vi "Send Actuator Setpoint.vi"(8 "error in (no error)":errorcluster, 10 "SlewFlag":bool, 11 "Model in":refnum<class "Model.lvclass">) -> (0 "error out":errorcluster, 3 "Model out":refnum<class "Model.lvclass">)   [LabVIEW 2016]
uses:
  Common_RT_FAILC/FAILC/FAILC.lvclass
  Modbus/DesktopModbus/DesktopModbus.lvclass
  Model.lvclass
  C:/CODE/ts_HPMT/Common_RT_ILC/ILC/ILC.lvclass
  C:/CODE/ts_HPMT/Common_RT_Modbus/IModbus/IModbus.lvclass
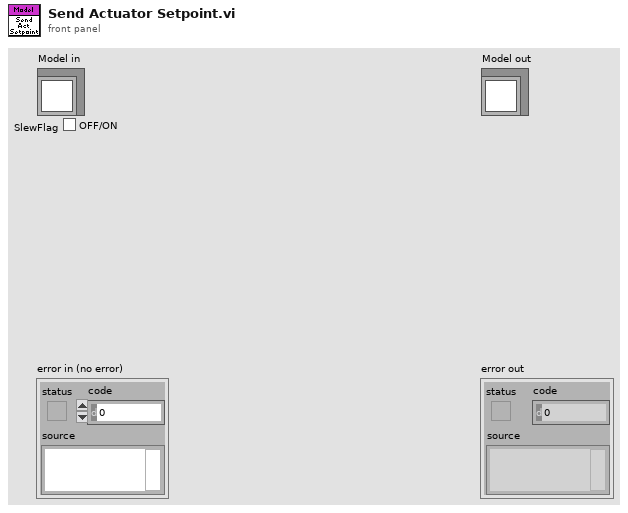
[diagram p1: front panel]
types:
  T1 = typedef "RTHPILC.lvlib/HPData.ctl" = cluster{"Constants":T2, "Command":T3, "Telemetry":T4, "Responses":T5, "Timings":T7}
  T2 = typedef "RTHPILC.lvlib/HPConstants.ctl" = cluster{"ID":i16}
  T3 = typedef "RTHPILC.lvlib/HPCommand.ctl" = cluster{"AxialSetPoint":i32, "LateralSetPoint":i32, "AxialBoosterValveGain":sgl, "LateralBoosterValveGain":sgl}
  T4 = typedef "RTHPILC.lvlib/HPTelemetry.ctl" = cluster{"ILCFault":bool, "BroadcastCounter":u8, "AxialLoadCellForce":sgl, "LateralLoadCellForce":sgl, "AxialBoosterValveGain":sgl, "LateralBoosterValveGain":sgl}
  T5 = typedef "RTHPILC.lvlib/HPResponses.ctl" = cluster{"BoosterValveGain":T6, "ReadBoosterValveGain":T6, "SetForce":T6, "ForceAndStatus":T6}
  T6 = typedef "RTModbus.lvlib/ExceptionCodes.ctl" = u16
  T7 = typedef "RTHPILC.lvlib/HPTimings.ctl" = cluster{"BroadcastSetForce":u32, "BoosterValveGain":u32, "FreezeSensorValues":u32, "ForceAndStatus":u32, "ReadBoosterValveGain":u32, "SetForce":u32}
  T8 = typedef "RTModbus.lvlib/TxFrame.ctl" = cluster{"Data":u8[], "WaitForTrigger":bool, "WaitForRx":u16, "TriggerIRQ":bool, "DelayMicroseconds":u16, "DelayMilliseconds":u16, "Timestamp":bool}
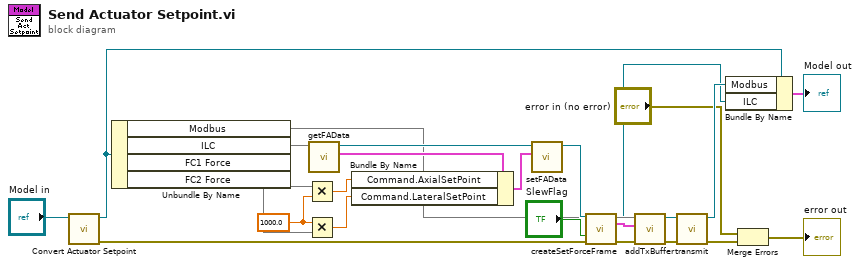
[diagram p0: block diagram]
diagram:
  w21 = 1000.0 ("y")
  n1 = call "Convert Actuator Setpoint.vi"("Model in"="Model in") -> ("error out"=w2:errorcluster, "Model out"=w3:refnum<class "Model.lvclass">)  [unwired: 9 in]
  n2 = Unbundle By Name(w3) -> ("Modbus"=w13, "ILC"=w16, "FC1 Force"=w23, "FC2 Force"=w20)
  n3 = Multiply(x=w23, y=w21) -> (x*y=w22:dbl)
  n4 = Multiply(x=w21, y=w20) -> (x*y=w19:dbl)
  n5 = call "getFAData.vi"("FAILC in"=w16) -> ("FAData"=w24:T1, "FAILC out"=w17:refnum<class "FAILC.lvclass">)  [unwired: 9 in]
  n6 = Bundle By Name(cluster=w24, "Command.AxialSetPoint"=w22, "Command.LateralSetPoint"=w19) -> (w18:T1)
  n7 = call "setFAData.vi"("FAData"=w18, "FAILC in"=w17) -> ("FAILC out"=w15:refnum<class "FAILC.lvclass">)  [unwired: 9 in]
  n8 = call-dynamic "createSetForceFrame.vi"("FAILC in"=w15, "SlewFlag"="SlewFlag", "error in (no error)"=w2) -> ("FAILC out"=w8:refnum<class "FAILC.lvclass">, "TxFrame"=w12:T8, "error out"=w11:errorcluster)  [unwired: 10 in]
  n9 = call-dynamic "addTxBuffer.vi"("error in (no error)"=w11, "TxFrame"=w12, "DesktopModbus in"=w13) -> ("error out"=w10:errorcluster, "DesktopModbus out"=w14:refnum<class "DesktopModbus.lvclass">)  [unwired: 7 in]
  n10 = call-dynamic "transmit.vi"("error in (no error)"=w10, "DesktopModbus in"=w14) -> ("error out"=w7:errorcluster, "DesktopModbus out"=w9:refnum<class "DesktopModbus.lvclass">)  [unwired: 8 in]
  n11 = Bundle By Name(cluster=w3, "Modbus"=w9, "ILC"=w8) -> (→"Model out":cluster{})
  n12 = Merge Errors("error in (no error)", w7) -> (→"error out":errorcluster)
